vi "InsideObstruction.vi"(8 "error in (no error)":errorcluster, 10 "point":cluster{"X":dbl, "Y":dbl}, 11 "Rectangle in":refnum<class "Rectangle.lvclass">) -> (0 "error out":errorcluster, 2 "inside":bool, 3 "Rectangle out":refnum<class "Rectangle.lvclass">)   [LabVIEW 2013, in "Rectangle.lvclass"]
uses:
  Rectangle.lvclass
  Rectangle.lvclass/Rectangle.ctl
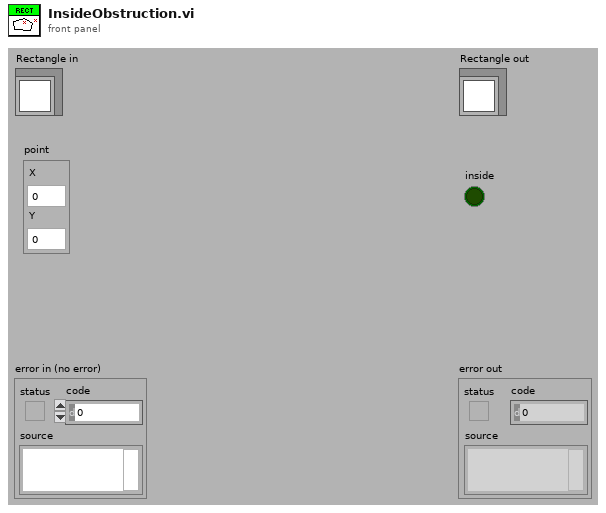
[diagram p1: front panel]
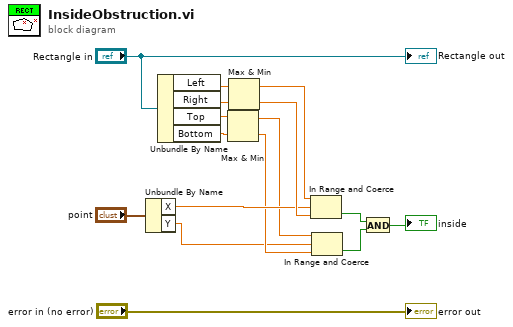
[diagram p0: block diagram]
diagram:
  n1 = Unbundle By Name("point") -> ("X"=w7:dbl, "Y"=w4:dbl)
  n2 = Unbundle By Name("Rectangle in") -> ("Left"=w13:dbl, "Right"=w12:dbl, "Top"=w11:dbl, "Bottom"=w10:dbl)
  n3 = Max & Min(x=w11, y=w10) -> (max(x,y)=w6:dbl, min(x,y)=w5:dbl)
  n4 = Max & Min(x=w13, y=w12) -> (max(x,y)=w9:dbl, min(x,y)=w8:dbl)
  n5 = In Range and Coerce(upper limit=w9, x=w7, lower limit=w8) -> (In Range?=w3:bool)  [unwired: 1 out]
  n6 = In Range and Coerce(upper limit=w6, x=w4, lower limit=w5) -> (In Range?=w2:bool)  [unwired: 1 out]
  n7 = And(x=w3, y=w2) -> (x .and. y?=→"inside":bool)
  "error out" <- "error in (no error)"
  "Rectangle out" <- "Rectangle in"
